vi "Excute.vi"(8 "error in (no error)":errorcluster, 11 "AfterDecorator in":refnum<class "AfterDecorator.lvclass">) -> (0 "error out":errorcluster, 3 "AfterDecorator out":refnum<class "AfterDecorator.lvclass">)   [LabVIEW 2014, in "AfterDecorator.lvclass"]
uses:
  AfterDecorator.lvclass
  Decorator_class/Decorator.lvclass
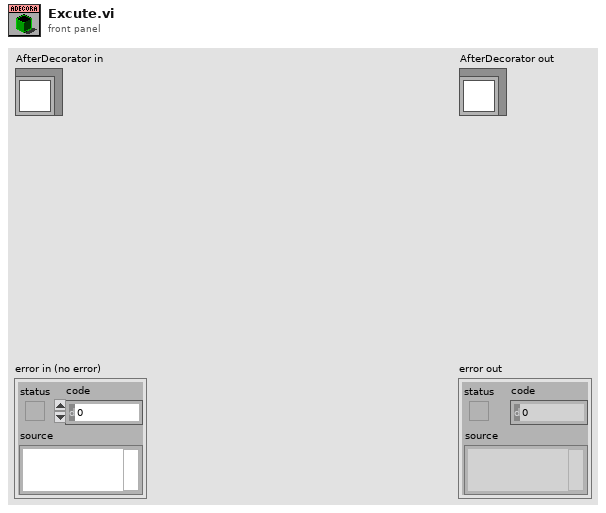
[diagram p1: front panel]
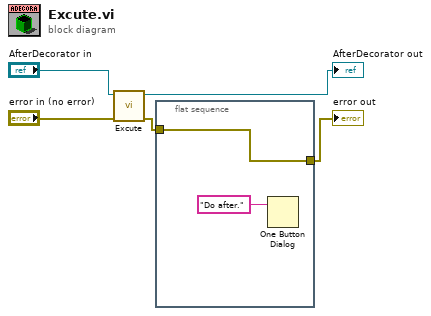
[diagram p0: block diagram]
diagram:
  n1 = call-parent "Excute.vi"("error in (no error)"="error in (no error)", "Decorator in"="AfterDecorator in") -> ("error out"=w2:errorcluster, "Decorator out"=→"AfterDecorator out":refnum<class "AfterDecorator.lvclass">)  [unwired: 8 in]
  n2 = flat-sequence {
    tunnel: [w6] -> w1
    tunnel: w2 -> [w6]
    frame #0 {
      n3 = One Button Dialog(message="Do after.") -> ()  [unwired: 1 in, 1 out]
    }
  }
  "error out" <- w1
